vi "LabView Control.vi"() -> ()   [LabVIEW 2011]
uses:
  <vilib>/DAQmx/read.llb/DAQmx Read (Analog DBL 1Chan 1Samp).vi
  <vilib>/DAQmx/create/channels.llb/DAQmx Create Channel (AI-Voltage-Basic).vi
  <vilib>/DAQmx/miscellaneous.llb/DAQmx Fill In Error Info.vi
panel:
  in  "frequency (1E+3)":dbl=1000.0 format="%.2p"
  in  "Save Data":bool
  in  "millisecond timer value":u32=300
  out "Voltage In":dbl(graph)
  in  "Stop":bool
  in  "amplitude (2.00)":dbl=0.01 format="%.2p"
  in  "waveform (sine)":i32(ring)=1 items=["Sine"=1, "Square"=2, "Triangle"=3, "Ramp Up"=4, "Noise"=1001]
  out "firmware revision":string
  out "instrument driver revision":string
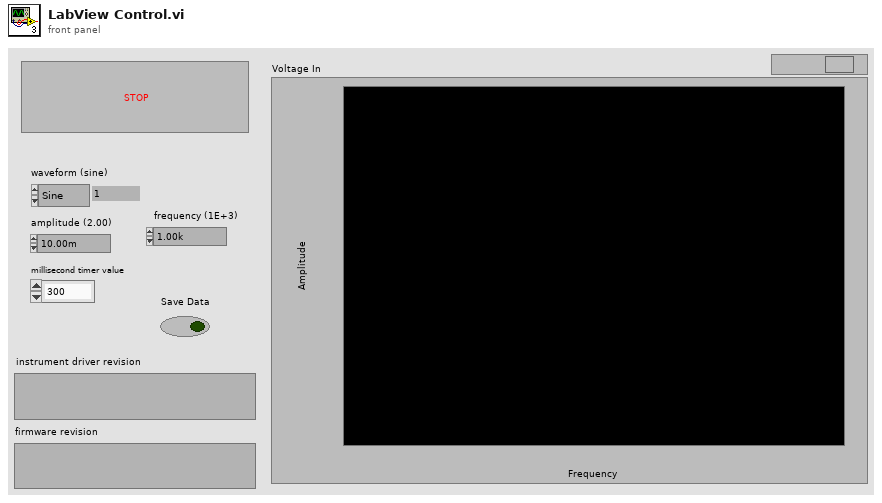
[diagram p1: front panel]
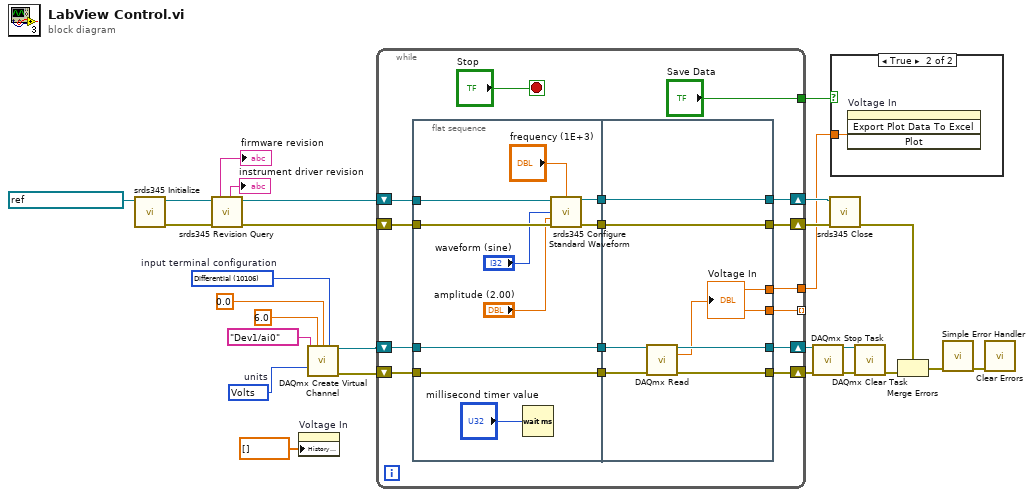
[diagram p0: block diagram]
diagram:
  w3 = 10106 items=["default"=-1, "RSE"=10083, "NRSE"=10078, "Differential"=10106, "Pseudodifferential"=12529]  # input terminal configuration
  w2 = 10348 items=["Volts"=10348, "From Custom Scale"=10065]  # units
  n1 = call <instrlib>:"srds345 Initialize.vi"("resource name (\"GPIB::14::INSTR\")"=refnum<k15> "GPIB0::20::INSTR" ("resource name (\"GPIB::14::INSTR\")")) -> ("error out"=w26:errorcluster, "instrument handle out"=w27:refnum<k15>)  [unwired: 9 in]
  n2 = call <instrlib>:"srds345 Revision Query.vi"("error in (no error)"=w26, "instrument handle"=w27) -> ("error out"=w24:errorcluster, "firmware revision"=→"firmware revision":string, "instrument driver revision"=→"instrument driver revision":string, "instrument handle out"=w25:refnum<k15>)  [unwired: 6 in]
  n3 = property on="Voltage In" class="WFChart (strict)"("History Data"=dbl[] []) -> ()  [unwired: 2 in, 2 out]
  n4 = call-poly <vilib>:"DAQmx Create Virtual Channel.vi"("maximum value"=6.0, "minimum value"=0.0, "input terminal configuration"=w3, "physical channels"=tag "Dev1/ai0", "units"=w2) -> ("task out"=w7:refnum<k21>, "error out"=w6:errorcluster)  [unwired: 9 in]
  n5 = while {
    tunnel: [w43] -> _ mode=indexing
    shift-right: [w39] -> w23
    shift-left: w24 -> [w41]
    shift-right: [w31] -> w21
    shift-left: w6 -> [w35]
    shift-right: [w37] -> w19
    shift-left: w25 -> [w42]
    shift-right: [w32] -> w22
    shift-left: w7 -> [w36]
    tunnel: ["Save Data"] -> w9
    tunnel: [w30] -> w11
    stop <- "Stop" stop-if-true
    n6 = flat-sequence {
      tunnel: w42 -> [w48]
      tunnel: w41 -> [w53]
      tunnel: [w50] -> w40
      tunnel: [w49] -> w38
      tunnel: w36 -> [w52]
      tunnel: w35 -> [w51]
      tunnel: [w52] -> w34
      tunnel: [w51] -> w33
      tunnel: [w60] -> w32
      tunnel: [w59] -> w31
      tunnel: [w54] -> w43
      tunnel: [w58] -> w39
      tunnel: w40 -> [w58]
      tunnel: [w57] -> w37
      tunnel: w38 -> [w57]
      tunnel: w34 -> [w56]
      tunnel: w33 -> [w55]
      tunnel: [w54] -> w30
      frame #0 {
        n7 = Wait (ms)(milliseconds to wait="millisecond timer value") -> ()  [unwired: 1 out]
        n8 = call <instrlib>:"srds345 Configure Standard Waveform.vi"("instrument handle"=w48, "frequency (1E+3)"="frequency (1E+3)", "waveform (sine)"="waveform (sine)", "amplitude (2.00)"="amplitude (2.00)", "error in (no error)"=w53) -> ("instrument handle out"=w49:refnum<k15>, "error out"=w50:errorcluster)  [unwired: 9 in]
      }
      frame #1 {
        n9 = call-poly <vilib>:"DAQmx Read.vi"("task/channels in"=w56, "error in"=w55) -> ("task out"=w60:refnum<k21>, "data"=w54:dbl, "error out"=w59:errorcluster)  [unwired: 11 in]
        "Voltage In" <- w54
      }
    }
  }
  n10 = call <vilib>:"DAQmx Stop Task.vi"("task/channels in"=w22, "error in"=w21) -> ("task out"=w18:refnum<k21>, "error out"=w17:errorcluster)  [unwired: 12 in]
  n11 = call <instrlib>:"srds345 Close.vi"("error in (no error)"=w23, "instrument handle"=w19) -> ("error out"=w15:errorcluster)  [unwired: 9 in]
  n12 = case shown="True" w9 {
    tunnel: w11 -> [_ w61]
    frame False {
    }
    frame True {
      n13 = invoke on="Voltage In" class="WFChart (strict)" method="Export Plot Data To Excel"("Plot"=w61) -> ()  [unwired: 3 in, 4 out]
    }
  }
  n14 = call <vilib>:"DAQmx Clear Task.vi"("task in"=w18, "error in"=w17) -> ("error out"=w16:errorcluster)  [unwired: 13 in]
  n15 = Merge Errors(w15, w16) -> (w14:errorcluster)
  n16 = call <vilib>:"Simple Error Handler.vi"("error in (no error)"=w14) -> ("error out"=w13:errorcluster)  [unwired: 4 in, 4 out]
  n17 = call <vilib>:"Clear Errors.vi"("error in (no error)"=w13) -> ()  [unwired: 6 in, 1 out]
